vi "test_debug_new_PID_v15_host_v1_SubVI.vi"(8 "error in":errorcluster, 11 "FPGA VI Reference In":T1) -> (0 "error out":errorcluster, 3 "FPGA VI Reference Out":T1)   [LabVIEW 2017]
uses:
  <vilib>/rvi/interface/nirviReadWriteControl/nirviReadWriteControl.xnode
  <vilib>/rvi/interface/Simulation/niFpgaSimulationCallBeginRW.vi
  <vilib>/rvi/errors/niLvFpgaAdjustHostInterfaceError.vi
  <vilib>/rvi/interface/nirviMethod/nirviMethod.xnode
  <vilib>/FPGAPlugInAG/Dynamic/niLvFpga_ReadFifo_Dynamic.vi
  <vilib>/rvi/errors/niLvFpgaMergeErrorWithErrorCode.vi
  NiFpgaLv.dll
  <vilib>/Utility/error.llb/Error Cluster From Error Code.vi
  <vilib>/Waveform/DWDTOps.llb/DWDT Append Digital Samples.vi
  <vilib>/FPGAPlugInAG/Dynamic/niLvFpga_ConfigureFifo_Dynamic.vi
  <vilib>/Utility/file.llb/Write To Spreadsheet File (DBL).vi
  RIG-SPECIFIC FILES/FPGA Refs/FPGA Ref.ctl
  <vilib>/Waveform/DWDTOps.llb/DWDT Binary U32 to Digital.vi
  <vilib>/Waveform/DWDTOps.llb/DWDT Binary U16 to Digital.vi
  Typedefs/Read Write Enum.ctl
panel:
  in  "Requested Depth 2":u32=2000000
  in  "Requested Depth":u32=2000000
  out "Numeric":i32
  in  "number_samples":u16=200
  out "error out":errorcluster
  out "read_value":u32[](graph)
  out "written_value":u32[](graph)
  out "written_data":digitalwaveform(graph)
  out "read_fifo2":u32
  out "read data":digitalwaveform(graph)
  in  "Stop Simulation 2":bool
  out "written/read data":digitalwaveform[](graph)
  out "error out 2":errorcluster
  out "complete frame 2":bool
  out "Elements Remaining 3":u32
  out "stop_loop 2":bool
  out "hi(x)":u32[](array[numeric])
  out "x_new":dbl[](array[numeric])
  out "num frames":u32
  out "Elements\nRemaining 2":u32
  out "stop_loop":bool
  in  "reset_graphs":bool
  in  "Save":bool
  out "x diff":dbl[](graph)
  out "x offset":dbl[](graph)
  out "x centroid ref":dbl[](graph)
  out "x centroid new":dbl[](graph)
  out "Actual Depth 2":u32
  out "Elements Remaining":u32
  out "Actual Depth":u32
  in  "number of frames":u32=5
  out "complete frame":bool
  out "booleans":digitalwaveform(graph)
  in  "Simulation Steps":u32=100
  in  "Stop Simulation":bool
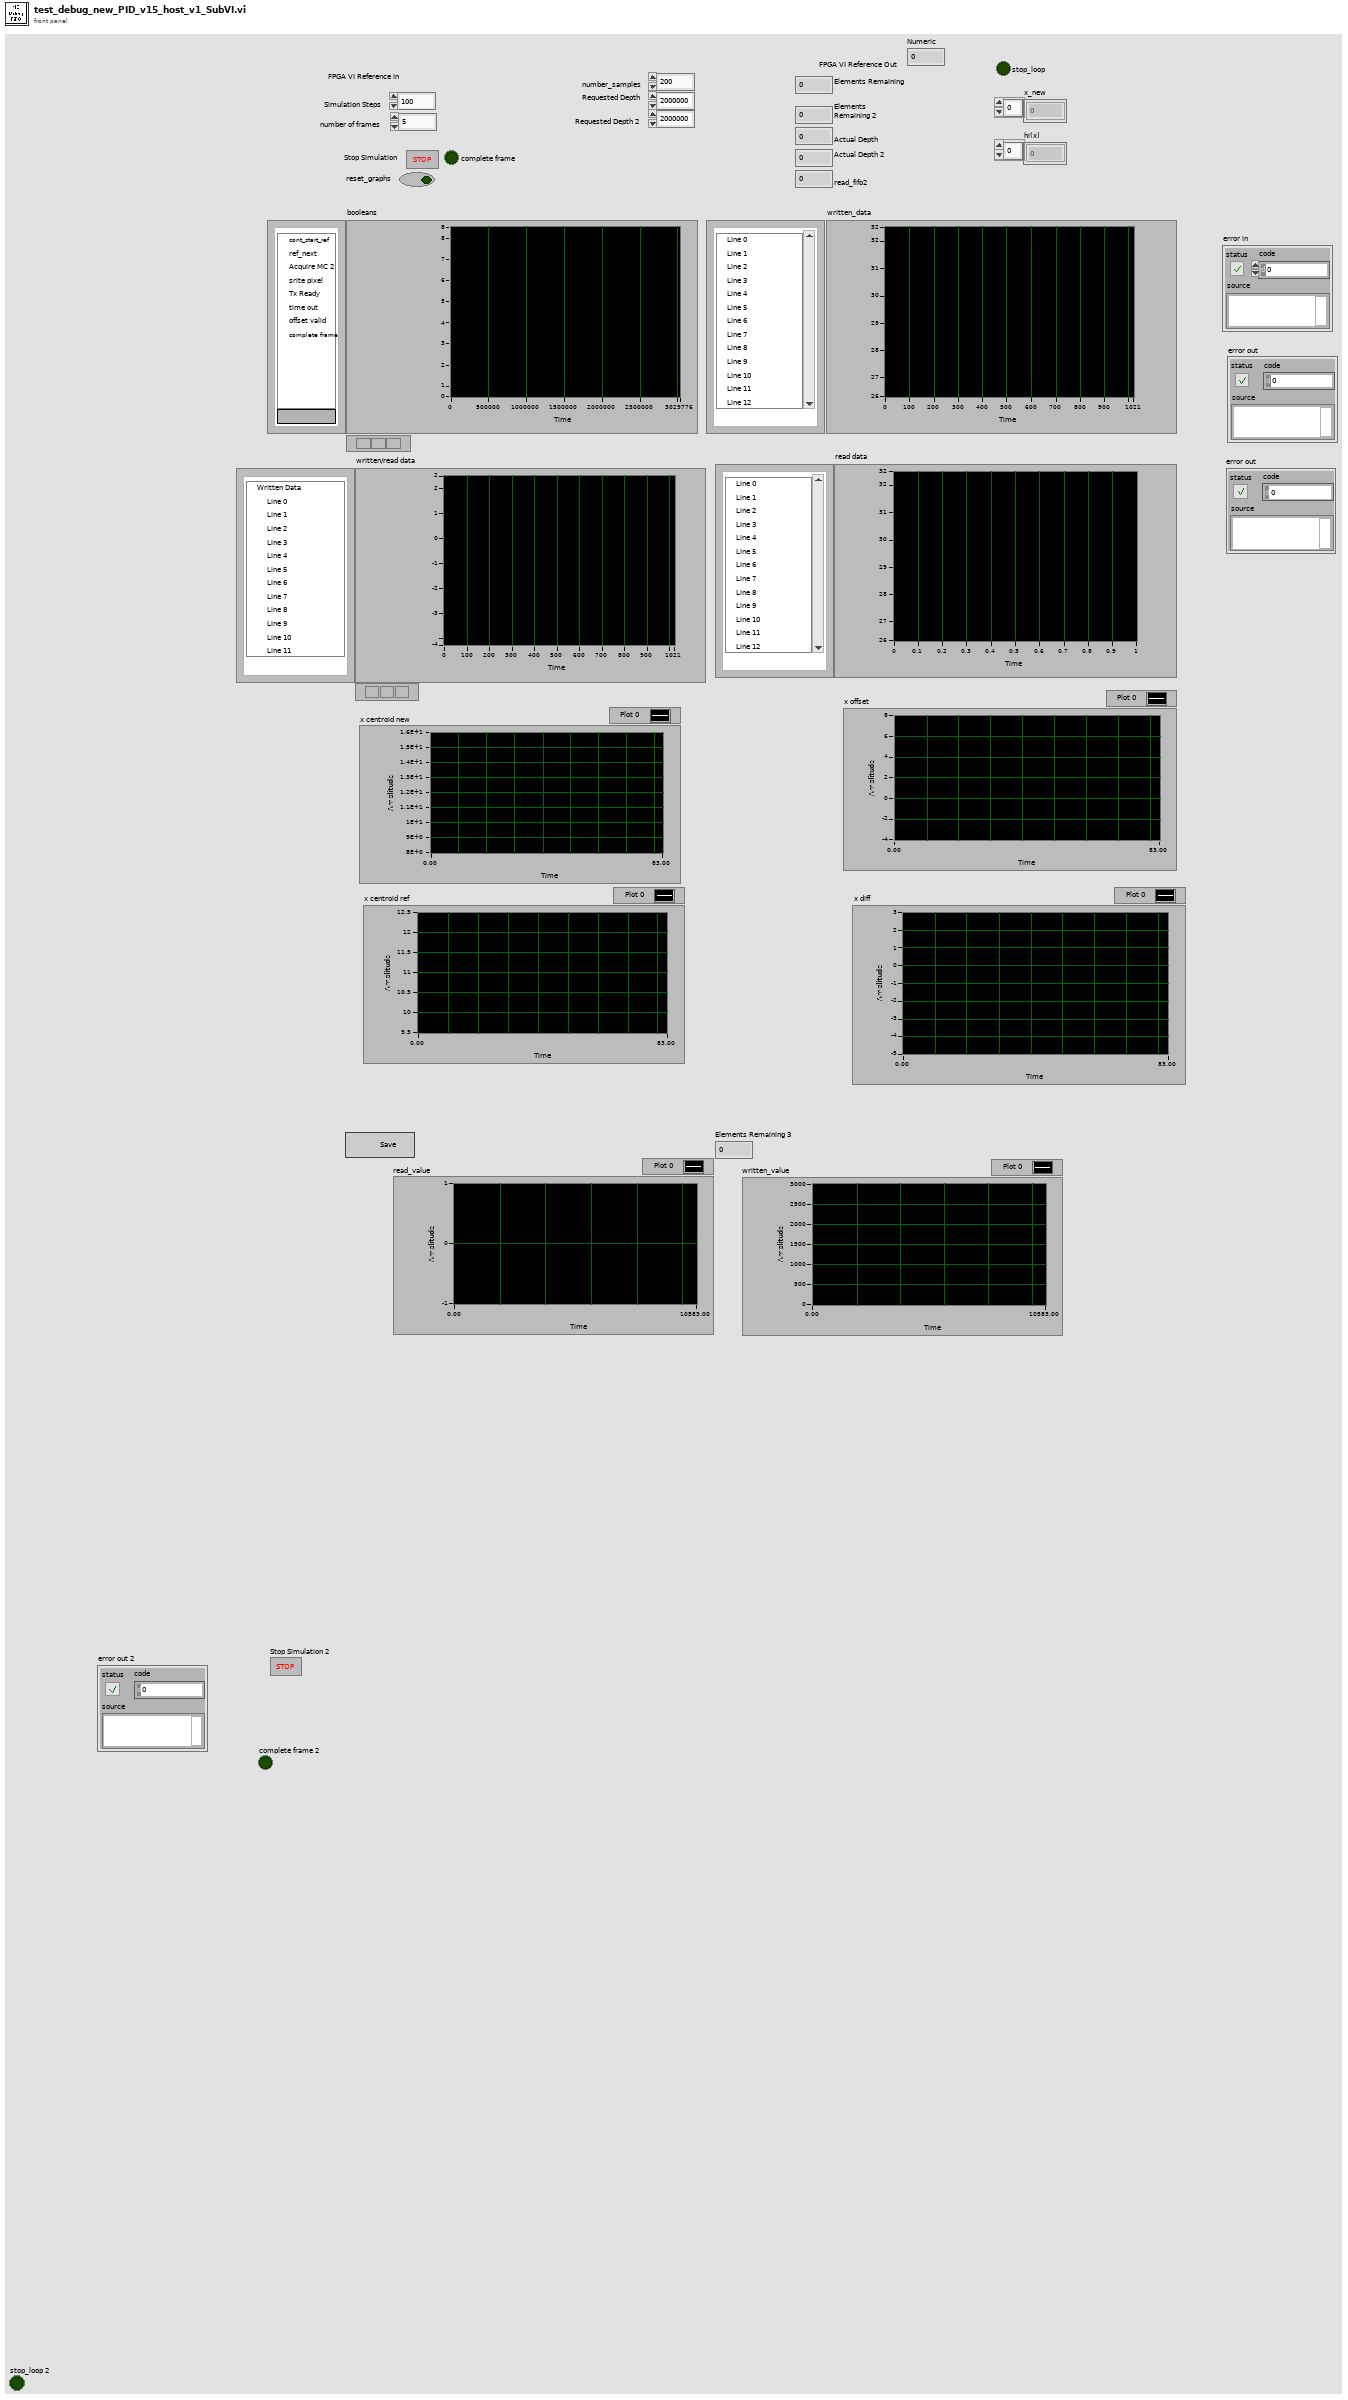
[diagram p1: front panel]
types:
  T1 = typedef "FPGA Ref.ctl" = refnum<k20>
  T2 = typedef "Read Write Enum.ctl" = enum16{"Read", "Write"}
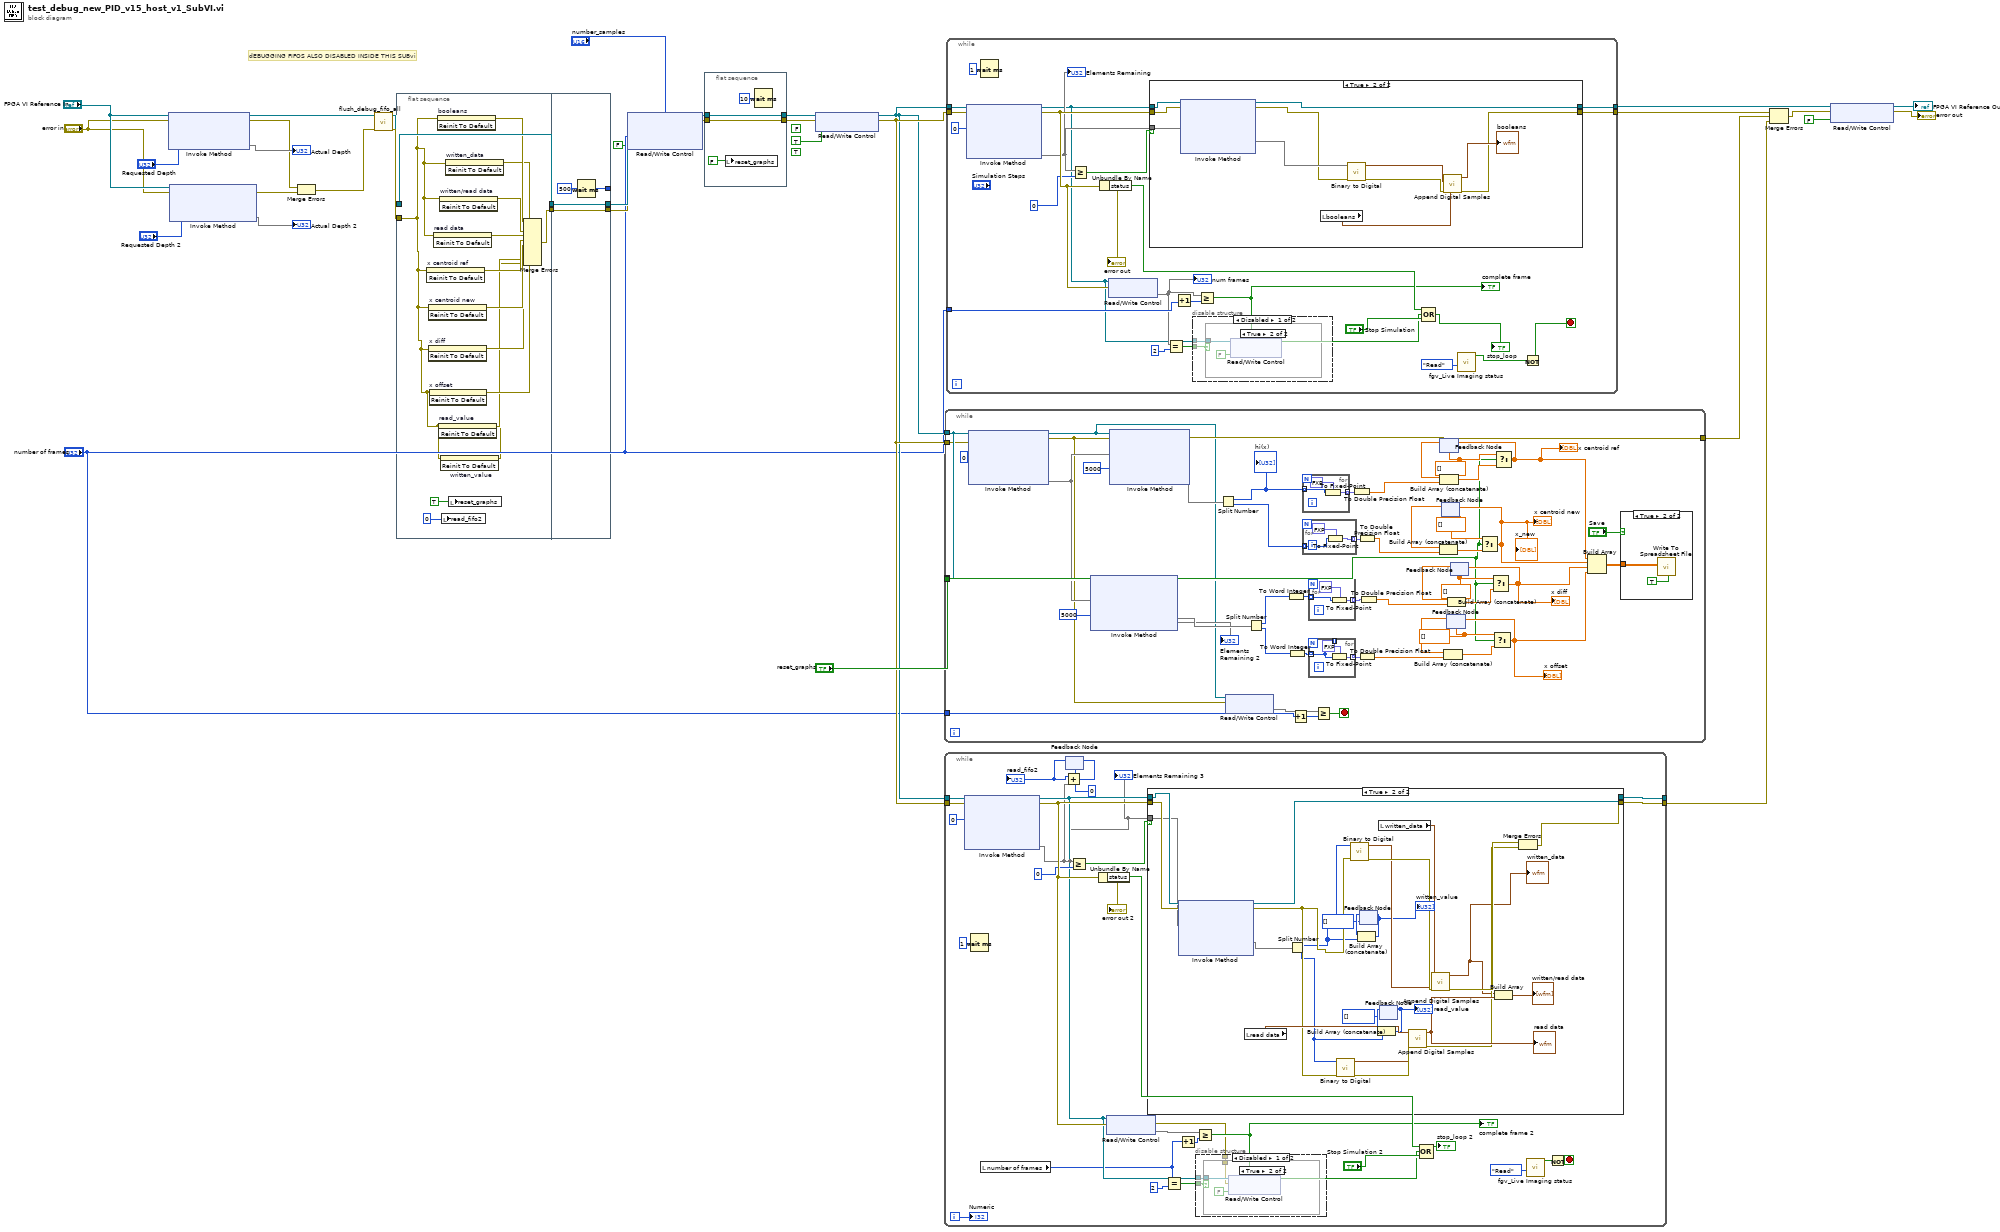
[diagram p0: block diagram]
diagram:
  (unwired) TRUE ("set_reference")
  (unwired) FALSE ("TX")
  # "dEBUGGING FIFOS ALSO DISABLED INSIDE THIS SUBvi"
  n1 = xnode "Invoke Method"("FPGA VI Reference In"="FPGA VI Reference In", "error in"="error in", "Requested Depth"="Requested Depth") -> ("FPGA VI Reference Out"=w25:T1, "error out"=w3:errorcluster, "Actual Depth"=→"Actual Depth")
  n2 = xnode "Invoke Method"("FPGA VI Reference In"="FPGA VI Reference In", "error in"="error in", "Requested Depth"="Requested Depth 2") -> ("error out"=w4:errorcluster, "Actual Depth"=→"Actual Depth 2")  [unwired: 1 out]
  n3 = Merge Errors(w3, w4) -> (w24:errorcluster)
  n4 = call "flush_debug_fifo_all.vi"("error in (no error)"=w24, "Refnum in"=w25) -> ("error out"=w30:errorcluster, "Refnum out"=w29:T1)  [unwired: 8 in]
  n5 = flat-sequence {
    tunnel: w30 -> [w38]
    tunnel: w29 -> [w49]
    tunnel: [w49] -> w35
    tunnel: [w41] -> w14
    tunnel: [w53] -> w16
    tunnel: [w52] -> w15
    tunnel: w35 -> [w53]
    tunnel: [w51] -> _
    tunnel: w14 -> [w52]
    frame #0 {
      n6 = invoke on="x centroid ref" class="WFGraph (strict)" method="Reinit To Default"(error in=w38) -> (error out=w45:errorcluster)  [unwired: 2 in, 2 out]
      n7 = invoke on="x centroid new" class="WFGraph (strict)" method="Reinit To Default"(error in=w38) -> (error out=w44:errorcluster)  [unwired: 2 in, 2 out]
      n8 = invoke on="x diff" class="WFGraph (strict)" method="Reinit To Default"(error in=w38) -> (error out=w43:errorcluster)  [unwired: 2 in, 2 out]
      n9 = invoke on="x offset" class="WFGraph (strict)" method="Reinit To Default"(error in=w38) -> (error out=w42:errorcluster)  [unwired: 2 in, 2 out]
      n10 = invoke on="read data" class="DigitalGraph (strict)" method="Reinit To Default"(error in=w38) -> (error out=w46:errorcluster)  [unwired: 2 in, 2 out]
      n11 = invoke on="booleans" class="DigitalGraph (strict)" method="Reinit To Default"(error in=w38) -> (error out=w48:errorcluster)  [unwired: 2 in, 2 out]
      n12 = invoke on="read_value" class="WFGraph (strict)" method="Reinit To Default"(error in=w38) -> (error out=w37:errorcluster)  [unwired: 2 in, 2 out]
      n13 = invoke on="written/read data" class="DigitalGraph (strict)" method="Reinit To Default"(error in=w38) -> (error out=w47:errorcluster)  [unwired: 2 in, 2 out]
      n14 = invoke on="written_value" class="WFGraph (strict)" method="Reinit To Default"(error in=w38) -> (error out=w36:errorcluster)  [unwired: 2 in, 2 out]
      n15 = local write "read_fifo2"(u32 0 ("read_fifo2")) -> ()
      n16 = invoke on="written_data" class="DigitalGraph (strict)" method="Reinit To Default"(error in=w38) -> (error out=w39:errorcluster)  [unwired: 2 in, 2 out]
      n17 = local write "reset_graphs"(TRUE ("reset_graphs")) -> ()
      n18 = Merge Errors(w48, w39, w47, w46, w45, w44, w43, w42, w37, w36) -> (w41:errorcluster)
    }
    frame #1 {
      n19 = Wait (ms)(milliseconds to wait=u32 500) -> (millisecond timer value=w51:u32)
    }
  }
  n20 = xnode "Read/Write Control"("FPGA VI Reference In"=w16, "error in"=w15, "number_samples"="number_samples", "num_frames_to_read"="number of frames", "contref(T)/spidata(F)"=FALSE) -> ("FPGA VI Reference Out"=w32:T1, "error out"=w31:errorcluster)
  n21 = flat-sequence {
    tunnel: [w57] -> w34
    tunnel: w32 -> [w57]
    tunnel: w31 -> [w56]
    tunnel: [w56] -> w33
    frame #0 {
      n22 = local write "reset_graphs"(FALSE ("reset_graphs")) -> ()
      n23 = Wait (ms)(milliseconds to wait=u32 10) -> ()  [unwired: 1 out]
    }
  }
  n24 = xnode "Read/Write Control"("FPGA VI Reference In"=w34, "error in"=w33, "debug_fifo_write"=TRUE) -> ("FPGA VI Reference Out"=w18:T1, "error out"=w19:errorcluster)
  n25 = while {
    tunnel: "reset_graphs" -> [_]
    tunnel: "reset_graphs" -> [w76]
    tunnel: w18 -> [w71]
    tunnel: w19 -> [w69]
    tunnel: [w68] -> w22
    tunnel: "number of frames" -> [w63]
    stop <- w61 stop-if-true
    w79 = dbl[] [] ("double precision float")
    w87 = dbl[] []
    w88 = dbl[] []
    w90 = dbl[] []
    n26 = xnode "Invoke Method"("FPGA VI Reference In"=w71, "error in"=w69, "Number of Elements"=u32 0) -> ("FPGA VI Reference Out"=w64:T1, "error out"=w65:errorcluster, "Elements Remaining"=w74)  [unwired: 1 in, 1 out]
    n27 = xnode "Invoke Method"("FPGA VI Reference In"=w71, "Number of Elements"=w74, "Timeout (ms)"=5000) -> ("Data"=w73:void[], "Elements Remaining"=→"Elements\nRemaining 2")  [unwired: 1 in, 2 out]
    n28 = xnode "Invoke Method"("FPGA VI Reference In"=w64, "error in"=w65, "Number of Elements"=w74, "Timeout (ms)"=5000) -> ("error out"=w68:errorcluster, "Data"=w75:void[])  [unwired: 2 out]
    n29 = Split Number(x=w75) -> (hi(x)=w105:u16[], lo(x)=w107:u16[])
    "hi(x)" <- w105
    n30 = xnode "Read/Write Control"("FPGA VI Reference In"=w64, "error in"=w65) -> ("num frames"=w66)  [unwired: 2 out]
    n31 = Split Number(x=w73) -> (hi(x)=w102:u16[], lo(x)=w101:u16[])
    n32 = To Word Integer(number=w102) -> (16bit integer=w78:i16[])
    n33 = To Word Integer(number=w101) -> (16bit integer=w77:i16[])
    n34 = Increment(x=w63) -> (x+1=w62:u32)
    n35 = for {
      tunnel: w105 -> [w117] mode=indexing
      tunnel: [w116] -> w104 mode=indexing
      n36 = To Fixed-Point(fixed-point type=fxp<+,32,16> 0.0 ("x_centroid_ref"), number=w117) -> (fixed-point=w116:fxp<+,32,16>)
    }
    n37 = for {
      tunnel: w107 -> [w120] mode=indexing
      tunnel: [w119] -> w106 mode=indexing
      n38 = To Fixed-Point(fixed-point type=fxp<+,32,16> 0.0 ("x_centroid_ref"), number=w120) -> (fixed-point=w119:fxp<+,32,16>)
    }
    n39 = for {
      tunnel: w78 -> [w112] mode=indexing
      tunnel: [w111] -> w103 mode=indexing
      n40 = To Fixed-Point(fixed-point type=fxp<+/-,16,8> 0.0 ("x-y"), number=w112) -> (fixed-point=w111:fxp<+/-,16,8>)
    }
    n41 = for {
      tunnel: w77 -> [w113] mode=indexing
      tunnel: [w115] -> w80 mode=indexing
      tunnel: [w113] -> _ mode=indexing
      n42 = To Fixed-Point(fixed-point type=fxp<+/-,16,8> 0.0 ("x-y"), number=w113) -> (fixed-point=w115:fxp<+/-,16,8>)
    }
    n43 = Greater Or Equal?(x=w66, y=w62) -> (x >= y?=w61:bool)
    n44 = To Double Precision Float(number=w104) -> (double precision float=w94:dbl[])
    n45 = To Double Precision Float(number=w106) -> (double precision float=w97:dbl[])
    n46 = To Double Precision Float(number=w80) -> (double precision float=w59:dbl[])
    n47 = To Double Precision Float(number=w103) -> (double precision float=w92:dbl[])
    n48 = feedback #1(w88) -> (w95:dbl[])
    n49 = Build Array (concatenate)(w95, w94) -> (w89:dbl[])
    n50 = feedback #2(w90) -> (w98:dbl[])
    n51 = Build Array (concatenate)(w98, w97) -> (w96:dbl[])
    n52 = feedback #3(w79) -> (w91:dbl[])
    n53 = Build Array (concatenate)(w91, w59) -> (w85:dbl[])
    n54 = feedback #4(w87) -> (w93:dbl[])
    n55 = Build Array (concatenate)(w93, w92) -> (w86:dbl[])
    n56 = Select(t=w90, s=w76, f=w96) -> (s? t:f=w83:dbl[])
    "x centroid new" <- w83
    "x_new" <- w83
    n57 = feedback-in #2(w83) -> ()
    n58 = Select(t=w87, s=w76, f=w86) -> (s? t:f=w82:dbl[])
    "x diff" <- w82
    n59 = feedback-in #4(w82) -> ()
    n60 = Select(t=w79, s=w76, f=w85) -> (s? t:f=w81:dbl[])
    "x offset" <- w81
    n61 = feedback-in #3(w81) -> ()
    n62 = Select(t=w88, s=w76, f=w89) -> (s? t:f=w84:dbl[])
    "x centroid ref" <- w84
    n63 = feedback-in #1(w84) -> ()
    n64 = Build Array(w84, w83, w82, w81) -> (w100:dbl[][])
    n65 = case shown="True" "Save" {
      tunnel: w100 -> [_ w109]
      frame False {
      }
      frame True {
        n66 = call-poly <vilib>:"Write To Spreadsheet File.vi"("transpose? (no:F)"=TRUE, "2D data"=w109) -> ()  [unwired: 6 in, 1 out]
      }
    }
  }
  n67 = while {
    tunnel: [w146] -> w17
    tunnel: [w147] -> _
    tunnel: w19 -> [w136]
    tunnel: w18 -> [w135]
    i -> [w125]
    stop <- w124 stop-if-true
    n68 = xnode "Invoke Method"("FPGA VI Reference In"=w135, "error in"=w136, "Number of Elements"=u32 0) -> ("FPGA VI Reference Out"=w137:T1, "error out"=w144:errorcluster, "Elements Remaining"=w132)  [unwired: 1 in, 1 out]
    "error out 2" <- w144
    "Elements Remaining 3" <- w132
    n69 = Wait (ms)(milliseconds to wait=u32 1) -> ()  [unwired: 1 out]
    n70 = local read "number of frames"() -> (w133:u32)
    n71 = feedback #5(u32 0) -> (w130:u32)
    "read_fifo2" <- w130
    n72 = Add(x=w130, y=w132) -> (x+y=w131:u32)
    n73 = feedback-in #5(w131) -> ()
    n74 = Greater Or Equal?(x=w132, y=u32 0) -> (x >= y?=w145:bool)
    n75 = Unbundle By Name(w144) -> ("status"=w143:bool)
    n76 = xnode "Read/Write Control"("FPGA VI Reference In"=w137, "error in"=w144) -> ("error out"=w127:errorcluster, "num frames"=w134)  [unwired: 1 out]
    n77 = case shown="True" w145 {
      tunnel: w137 -> [w157 w181]
      tunnel: [w157 w176] -> w147
      tunnel: w144 -> [w156 w180]
      tunnel: [w156 w173] -> w146
      tunnel: w132 -> [_ w179]
      frame False {
      }
      frame True {
        n78 = xnode "Invoke Method"("FPGA VI Reference In"=w181, "error in"=w180, "Number of Elements"=w179) -> ("FPGA VI Reference Out"=w176:T1, "error out"=w170:errorcluster, "Data"=w183:void[])  [unwired: 1 in, 1 out]
        n79 = local read "read data"() -> (w177:digitalwaveform)
        n80 = Split Number(x=w183) -> (hi(x)=w165:u16[], lo(x)=w159:u16[])
        n81 = call-poly <vilib>:"Binary to Digital.vi"("error in (no error)"=w170, "binary array"=w159) -> ("error out"=w171:errorcluster, "digital waveform"=w168:digitalwaveform)  [unwired: 8 in]
        n82 = call-poly <vilib>:"Binary to Digital.vi"("error in (no error)"=w170, "binary array"=w165) -> ("error out"=w172:errorcluster, "digital waveform"=w169:digitalwaveform)  [unwired: 8 in]
        n83 = feedback #6(u32[] []) -> (w164:u32[])
        n84 = Build Array (concatenate)(w164, w165) -> (w162:u32[])
        "written_value" <- w162
        n85 = feedback-in #6(w162) -> ()
        n86 = local read "written_data"() -> (w166:digitalwaveform)
        n87 = feedback #7(u32[] []) -> (w161:u32[])
        n88 = Build Array (concatenate)(w161, w159) -> (w158:u32[])
        "read_value" <- w158
        n89 = feedback-in #7(w158) -> ()
        n90 = call-poly <vilib>:"Append Digital Samples.vi"("error in (no error)"=w171, "digital waveform B"=w168, "digital waveform A"=w177) -> ("error out"=w174:errorcluster, "digital waveform out"=w178:digitalwaveform)  [unwired: 7 in]
        "read data" <- w178
        n91 = call-poly <vilib>:"Append Digital Samples.vi"("error in (no error)"=w172, "digital waveform B"=w169, "digital waveform A"=w166) -> ("error out"=w175:errorcluster, "digital waveform out"=w167:digitalwaveform)  [unwired: 7 in]
        "written_data" <- w167
        n92 = Build Array(w167, w178) -> (→"written/read data":digitalwaveform[])
        n93 = Merge Errors(w175, w174) -> (w173:errorcluster)
      }
    }
    n94 = Equal?(x=w133, y=u32 2) -> (x = y?=w138:bool)
    n95 = Increment(x=w133) -> (x+1=w141:u32)
    n96 = disable-structure shown="Disabled" {
      disable-tunnel: w138 -> [w152 _]
      disable-tunnel: w137 -> [w151 _]
      disable-tunnel: w127 -> [w150 _]
      frame Disabled {
        n97 = case shown="True" w152 {
          tunnel: w151 -> [_ w155]
          tunnel: w150 -> [_ w153]
          frame False {
          }
          frame True {
            n98 = xnode "Read/Write Control"("FPGA VI Reference In"=w155, "error in"=w153, "set_reference"=FALSE) -> ()  [unwired: 2 out]
          }
        }
      }
      frame Enabled {
      }
    }
    n99 = Greater Or Equal?(x=w134, y=w141) -> (x >= y?=w142:bool)
    "complete frame 2" <- w142
    n100 = Compound Arithmetic op=OR(w143, w142, "Stop Simulation 2") -> (→"stop_loop 2":bool)
    n101 = call "fgv_Live Imaging status.vi"("Function"=Read_Write_Enum."Read") -> ("Live Imaging?"=w122:bool)  [unwired: 9 in, 1 out]
    n102 = Not(x=w122) -> (.not. x?=w124:bool)
    "Numeric" <- w125
  }
  n103 = while {
    tunnel: w18 -> [w206]
    tunnel: w19 -> [w205]
    tunnel: [w200] -> w21
    tunnel: [w201] -> w26
    tunnel: "number of frames" -> [w196]
    stop <- w186 stop-if-true
    n104 = xnode "Invoke Method"("FPGA VI Reference In"=w206, "error in"=w205, "Number of Elements"=u32 0) -> ("FPGA VI Reference Out"=w188:T1, "error out"=w198:errorcluster, "Elements Remaining"=w192)  [unwired: 1 in, 1 out]
    "error out" <- w198
    "Elements Remaining" <- w192
    n105 = Wait (ms)(milliseconds to wait=u32 1) -> ()  [unwired: 1 out]
    n106 = Greater Or Equal?(x=w192, y=u32 0) -> (x >= y?=w199:bool)
    n107 = Unbundle By Name(w198) -> ("status"=w197:bool)
    n108 = xnode "Read/Write Control"("FPGA VI Reference In"=w188, "error in"=w198) -> ("num frames"=w191)  [unwired: 2 out]
    "num frames" <- w191
    n109 = case shown="True" w199 {
      tunnel: w188 -> [w212 w218]
      tunnel: [w212 w223] -> w201
      tunnel: w198 -> [w211 w217]
      tunnel: [w211 w213] -> w200
      tunnel: w192 -> [_ w216]
      frame False {
      }
      frame True {
        n110 = xnode "Invoke Method"("FPGA VI Reference In"=w218, "error in"=w217, "Number of Elements"=w216) -> ("FPGA VI Reference Out"=w223:T1, "error out"=w214:errorcluster, "Data"=w221:void[])  [unwired: 1 in, 1 out]
        n111 = local read "booleans"() -> (w222:digitalwaveform)
        n112 = call-poly <vilib>:"Binary to Digital.vi"("error in (no error)"=w214, "binary array"=w221) -> ("error out"=w215:errorcluster, "digital waveform"=w220:digitalwaveform)  [unwired: 8 in]
        n113 = call-poly <vilib>:"Append Digital Samples.vi"("error in (no error)"=w215, "digital waveform B"=w220, "digital waveform A"=w222) -> ("error out"=w213:errorcluster, "digital waveform out"=→"booleans":digitalwaveform)  [unwired: 7 in]
      }
    }
    n114 = Equal?(x=w191, y=u32 2) -> (x = y?=w189:bool)
    n115 = Increment(x=w196) -> (x+1=w194:u32)
    n116 = disable-structure shown="Disabled" {
      disable-tunnel: w189 -> [w208 _]
      disable-tunnel: w188 -> [w207 _]
      frame Disabled {
        n117 = case shown="True" w208 {
          tunnel: w207 -> [_ w210]
          frame False {
          }
          frame True {
            n118 = xnode "Read/Write Control"("FPGA VI Reference In"=w210, "set_reference"=FALSE) -> ()  [unwired: 1 in, 2 out]
          }
        }
      }
      frame Enabled {
      }
    }
    n119 = Greater Or Equal?(x=w191, y=w194) -> (x >= y?=w195:bool)
    "complete frame" <- w195
    n120 = Compound Arithmetic op=OR(w197, w195, "Stop Simulation") -> (→"stop_loop":bool)
    n121 = call "fgv_Live Imaging status.vi"("Function"=Read_Write_Enum."Read") -> ("Live Imaging?"=w184:bool)  [unwired: 9 in, 1 out]
    n122 = Not(x=w184) -> (.not. x?=w186:bool)
  }
  n123 = Merge Errors(w21, w22, w17) -> (w20:errorcluster)
  n124 = xnode "Read/Write Control"("FPGA VI Reference In"=w26, "error in"=w20, "debug_fifo_write"=FALSE) -> ("FPGA VI Reference Out"=→"FPGA VI Reference Out":T1, "error out"=→"error out":errorcluster)
